vi "Set Timing from wash step.vi"(8 "error in (no error)":errorcluster, 10 "Car Wash  Steps":T1, 11 "Car Wash Controller Actor in":refnum<class "Car Wash Controller Actor.lvclass">) -> (0 "error out":errorcluster, 3 "Car Wash Controller Actor out":refnum<class "Car Wash Controller Actor.lvclass">)   [LabVIEW 2019]
uses:
  Simulated Wash Display Console Actor/Simulated Wash Display Console Actor Messages/Update Time Remaining Msg/Update Time Remaining Msg.lvclass
  Car Wash Controller Actor.lvclass
  C:/Program Files (x86)/National Instruments/LabVIEW 2019/vi.lib/ActorFramework/Actor/Actor.lvclass
  <vilib>/ActorFramework/Message Enqueuer/Message Enqueuer.lvclass
  Sim Entry Console Actor/Sim Entry Console Actor/Wash steps selection -Buttons.ctl
  Sim Entry Console Actor/Sim Entry Console Actor/Simulated Entry Console Actor.lvclass
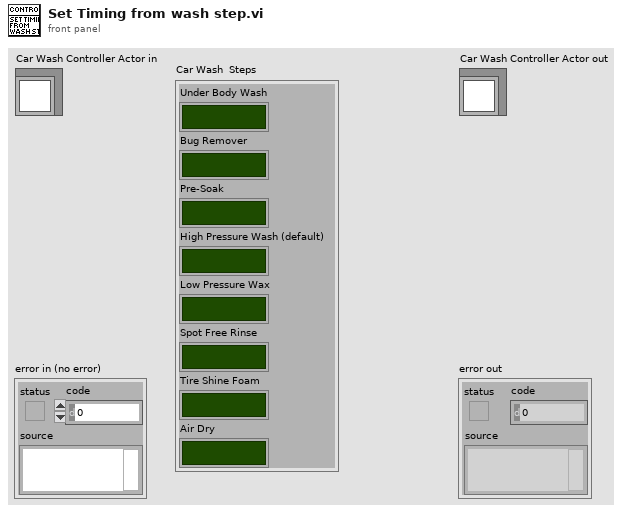
[diagram p1: front panel]
types:
  T1 = typedef "Simulated Entry Console Actor.lvlib/Simulated Entry Console Actor.lvclass/Wash steps selection -Buttons.ctl" = cluster{"Under Body Wash":bool, "Bug Remover":bool, "Pre-Soak":bool, "High Pressure Wash (default)":bool, "Low Pressure Wax":bool, "Spot Free Rinse":bool, "Tire Shine Foam":bool, "Air Dry":bool}
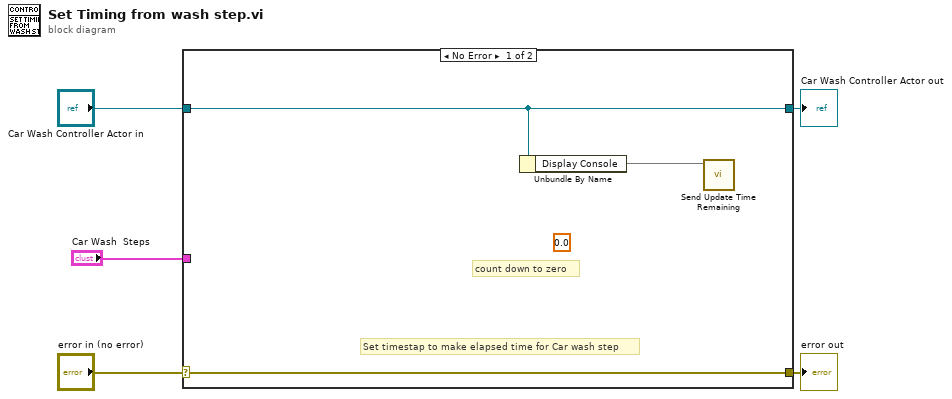
[diagram p0: block diagram]
diagram:
  n1 = case shown="No Error" "error in (no error)" {
    selector: "error in (no error)" -> [w8 w10]
    tunnel: [w8 w10] -> w4
    tunnel: [w7 w9] -> w2
    tunnel: "Car Wash Controller Actor in" -> [w7 w9]
    tunnel: "Car Wash  Steps" -> [_ _]
    frame No Error {
      (unwired) 0.0 ("Timing")
      # "count down to zero"
      # "Set timestap to make elapsed time for Car wash step"
      n2 = Unbundle By Name(w7) -> ("Display Console"=w6)
      n3 = call "Send Update Time Remaining.vi"("Message Enqueuer"=w6) -> ()  [unwired: 9 in, 2 out]
    }
    frame Error {
    }
  }
  "error out" <- w4
  "Car Wash Controller Actor out" <- w2
